vi "Data_Save_summary.vi"(8 "Data in":T1, 11 "AllControls In":T2) -> (2 "data":string[](array[string]), 3 "dup path":path)   [LabVIEW 2017]
uses:
  Ctrls/AllControls.ctl
  Ctrls/CSV_Data.ctl
  Ctrls/PathChoose.ctl
  <vilib>/Utility/file.llb/Write Delimited Spreadsheet (string).vi
  <vilib>/Utility/file.llb/Read Delimited Spreadsheet (string).vi
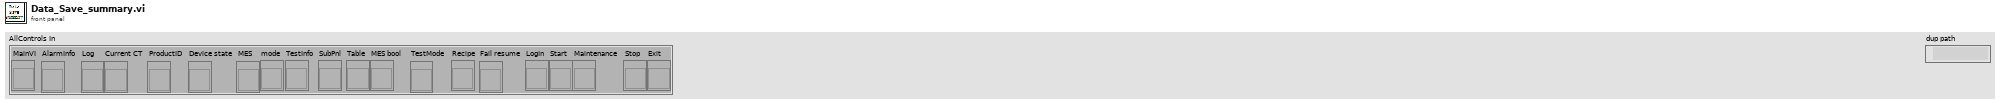
[diagram p1: front panel]
types:
  T1 = typedef "CSV_Data.ctl" = cluster{"Version":cluster{"SC_Version":string, "VP_Version":string}, "SN":string, "Table":string[][], "Count":cluster{"Total":i32, "OK":i32, "NG":i32, "Yield":dbl}, "Start Time":timestamp, "daemon reference":refnum<k5>, "CT":dbl, "Config":string[][], "OK/NG":bool, "Station ID":string, "MES DDM SN":string, "MES PCBA SN":string, "Retest":string, "Lux":string, "VOT":cluster{"Initial brightness":string, "Mean uniformity":string, "Uniformity_Deviation":string, "Adjusted brightness":string, "Mean_Adjusted":string, "Deviation_Adjusted":string, "Reflection":string, "Result":bool}, "SKU":string, "Plate_Diameter":string, "Alarm":string}
  T2 = typedef "AllControls.ctl" = cluster{"MainVI":refnum<vi>, "AlarmInfo":refnum<vi>, "Log":refnum<vi>, "Current CT":refnum<vi>, "ProductID":refnum<vi>, "Device state":refnum<vi>, "MES":refnum<vi>, "mode":refnum<vi>, "TestInfo":refnum<vi>, "SubPnl":refnum<vi>, "Table":refnum<vi>, "MES bool":refnum<vi>, "TestMode":refnum<vi>, "Recipe":refnum<vi>, "Fail resume":refnum<vi>, "LogIn":refnum<vi>, "Start":refnum<vi>, "Maintenance":refnum<vi>, "Stop":refnum<vi>, "Exit":refnum<vi>}
  T3 = typedef "PathChoose.ctl" = enum16{"OperatorLog", "AutoRunLog", "AlmLog", "TestData", "AllTestData", "backup_nvm", "backup_before_flashing"}
  T4 = enum16{"open", "replace", "create", "open or create", "replace or create", "replace or create with confirmation"}
  T5 = typedef "TesterInfo.ctl" = cluster{"Station Name":string, "Station Code":string, "ES NO.":string, "Tester ID":string, "PassMark Revision":string, "Rig ID":string, "682_Tool_Repeat":string, "Project Name":string, "FFTesterPath":path, "Enable_User":bool, "Mode":enum16{"682"}, "Fail_resume_mode":bool}
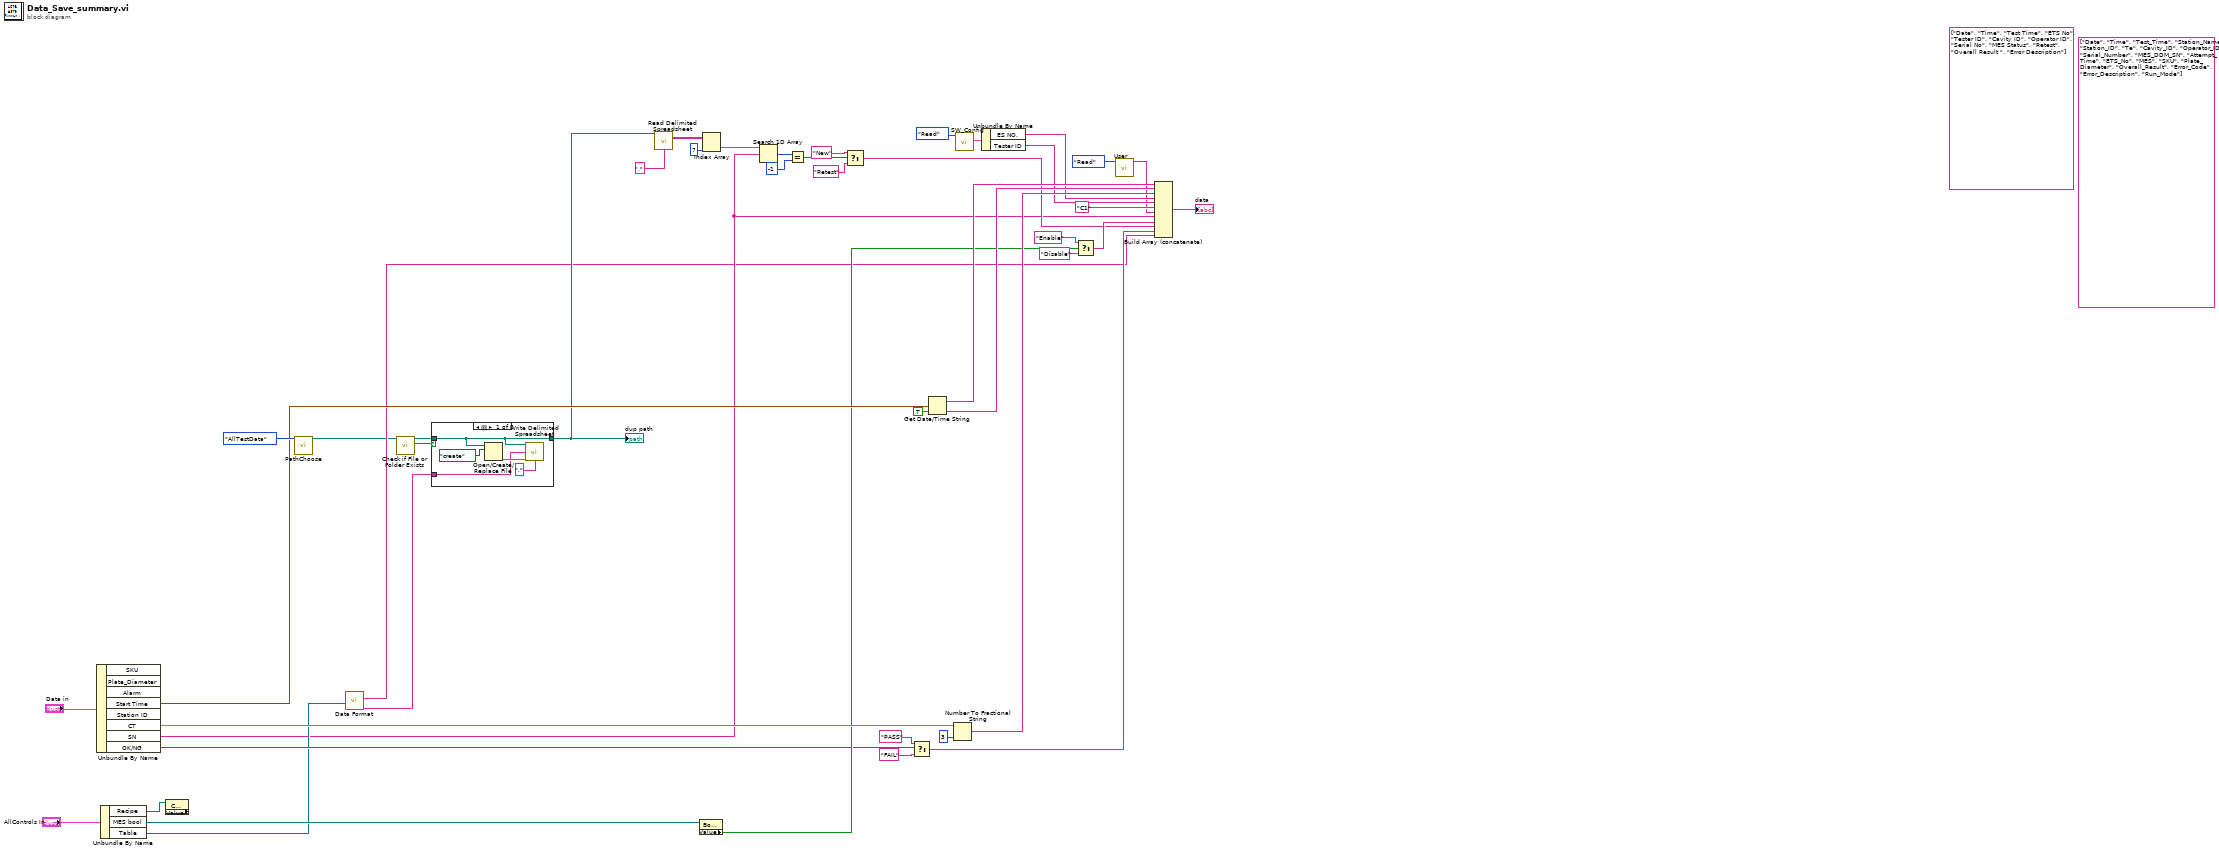
[diagram p0: block diagram]
diagram:
  (unwired) string[] ["Date", "Time", "Test Time", "ETS No", "Tester ID", "Cavity ID", "Operator ID", "Serial No", "MES Status", "Retest", "Overall Result ", "Error Description"] ("title")
  (unwired) string[] ["Date", "Time", "Test_Time", "Station_Name", "Station_ID", "Te", "Cavity_ID", "Operator_ID", "Serial_Number", "MES_DDM_SN", "Attempt_Time", "ETS_No", "MES", "SKU", "Plate_Diameter", "Overall_Result", "Error_Code", "Error_Description", "Run_Mode"]
  n1 = Unbundle By Name("Data in") -> ("Start Time"=w32:timestamp, "CT"=w39:dbl, "SN"=w4:string, "OK/NG"=w17:bool)  [unwired: 4 out]
  n2 = Unbundle By Name("AllControls In") -> ("Recipe"=w34:refnum<vi>, "MES bool"=w37:refnum<vi>, "Table"=w16:refnum<vi>)
  n3 = property class="CmbBox" props=["Value"](reference=w34) -> ()  [unwired: 1 in, 3 out]
  n4 = call "PathChoose.vi"(11:PathChoose."AllTestData") -> ("Path_Out"=w1:path)  [unwired: 10 in]
  n5 = call "Data Format.vi"("Table"=w16) -> ("title"=w33:string[], "Data"=w3:string[])  [unwired: 9 in]
  n6 = call <vilib>:"Check if File or Folder Exists.vi"("path"=w1) -> ("file or folder exists?"=w43:bool, "dup path"=w42:path)  [unwired: 8 in, 1 out]
  n7 = case shown="假" w43 {
    tunnel: w42 -> [w49 w52]
    tunnel: [w49 w52] -> w15
    tunnel: w33 -> [w47 _]
    frame False {
      n8 = Open/Create/Replace File(file path (use dialog)=w49, operation (0:open)=T4."create") -> (error out=w48:errorcluster)  [unwired: 4 in, 2 out]
      n9 = call-poly <vilib>:"Write Delimited Spreadsheet.vi"("file path (dialog if empty)"=w49, "1D data"=w47, "error in (no error)"=w48, "delimiter (\\t)"="," ("delimiter (\\t)")) -> ()  [unwired: 10 in, 2 out]
    }
    frame True {
    }
  }
  "dup path" <- w15
  n10 = call-poly <vilib>:"Read Delimited Spreadsheet.vi"("file path (dialog if empty)"=w15, "delimiter (\\t)"="," ("delimiter (\\t)")) -> ("all rows"=w13:string[][])  [unwired: 8 in, 5 out]
  n11 = property class="Bool (严格)"(reference=w37) -> ("Value"=w19:bool)  [unwired: 1 in, 2 out]
  n12 = Index Array(array=w13, index (col)=7 ("disabled index (col)")) -> (element=w11:string[])  [unwired: 1 in]
  n13 = Search 1D Array(1D array=w11, element=w4) -> (index of element=w10:i32)  [unwired: 1 in]
  n14 = Equal?(x=w10, y=-1) -> (x = y?=w8:bool)
  n15 = Select(t="New", s=w8, f="Retest") -> (s? t:f=w5:string)
  n16 = Select(t="PASS" ("真字符串"), s=w17, f="FAIL" ("假字符串")) -> (s? t:f=w18:string)
  n17 = Get Date/Time String(seconds (now)=w32, want seconds? (F)=TRUE ("需要秒？(F)")) -> (date string=w31:string, time string=w30:string)  [unwired: 1 in]
  n18 = Number To Fractional String(number=w39, precision (6)=i16 3 ("精度(6)")) -> (F-format string=w29:string)  [unwired: 2 in]
  n19 = call "SW_Config.vi"("Step"=enum16{"Initial", "Write", "Read"}."Read") -> ("SW Config out"=w27:T5)  [unwired: 9 in, 1 out]
  n20 = Unbundle By Name(w27) -> ("ES NO."=w26:string, "Tester ID"=w25:string)
  n21 = Select(t="Enable" ("element"), s=w19, f="Disable") -> (s? t:f=w20:string)
  n22 = call "User.vi"("Step"=enum16{"Initial", "Write", "Read"}."Read") -> ("User out"=w23:string)  [unwired: 9 in, 1 out]
  n23 = Build Array (concatenate)(w31, w30, w29, w26, w25, "C1" ("element"), w23, w4, w20, w5, w18, w3) -> (→"data":string[])
